vi "digital password.vi"() -> ()   [LabVIEW 2021]
panel:
  out "String":string
  out "String 3":string
  out "Password":string
  out "Slide":u8(slide) scale=0.0..100.0
  in  "Password":T1
  # "1"
  # "2"
  # "3"
  # "4"
  # "5"
  # "6"
  # "7"
  # "8"
  # "9"
  # "0"
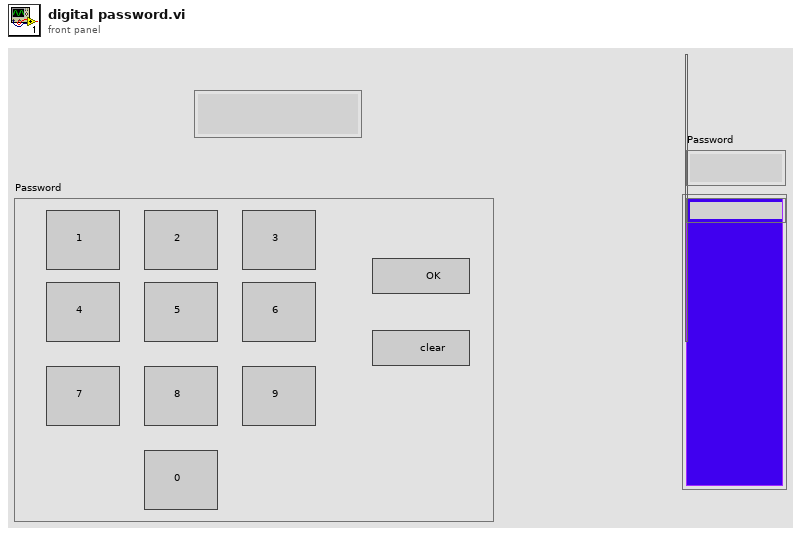
[diagram p1: front panel]
types:
  T1 = cluster{"Blank Button":bool, "Blank Button 2":bool, "Blank Button 3":bool, "Blank Button 4":bool, "Blank Button 5":bool, "Blank Button 6":bool, "Blank Button 7":bool, "Blank Button 8":bool, "Blank Button 9":bool, "Blank Button 10":bool, "OK Button":bool, "Refresh Button":bool}
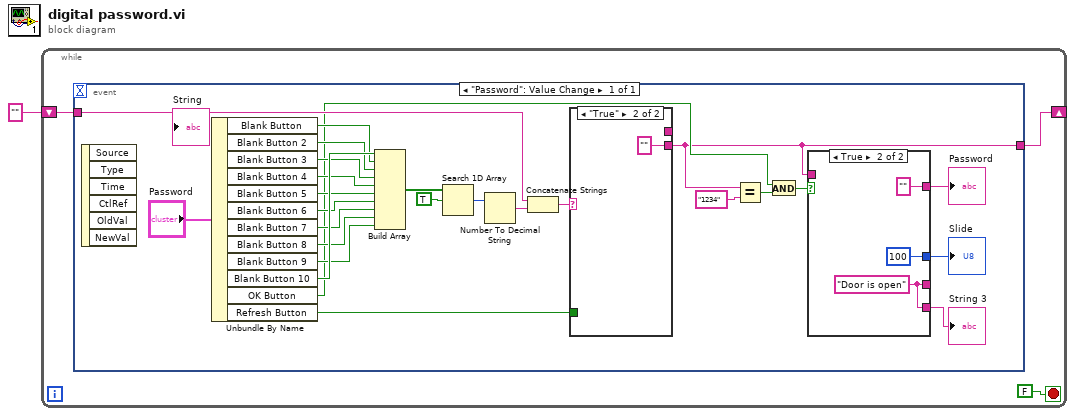
[diagram p0: block diagram]
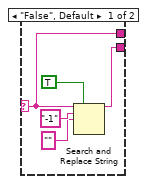
[diagram p2: hidden frame]
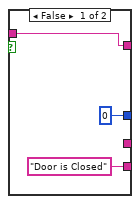
[diagram p3: hidden frame]
diagram:
  n1 = while {
    shift-right: [w3] -> _
    shift-left: "" -> [w2]
    stop <- FALSE stop-if-true
    n2 = event shown="[0] \"Password\": Value Change" {
      selector: _ -> [_]
      dyn-events: _ -> [_]
      timeout: _ -> [_]
      tunnel: [w5] -> w3
      tunnel: w2 -> [w15]
      event "Password": Value Change {
        n3 = event-data() -> ()  [unwired: 1 in, 6 out]
        n4 = Unbundle By Name("Password") -> ("Blank Button"=w28:bool, "Blank Button 2"=w27:bool, "Blank Button 3"=w26:bool, "Blank Button 4"=w25:bool, "Blank Button 5"=w24:bool, "Blank Button 6"=w23:bool, "Blank Button 7"=w22:bool, "Blank Button 8"=w21:bool, "Blank Button 9"=w20:bool, "Blank Button 10"=w29:bool, "OK Button"=w11:bool, "Refresh Button"=w7:bool)
        n5 = Build Array(w29, w28, w27, w26, w25, w24, w23, w22, w21, w20) -> (w18:bool[])
        n6 = Search 1D Array(1D array=w18, element=TRUE) -> (index of element=w19:i32)  [unwired: 1 in]
        n7 = Number To Decimal String(number=w19) -> (decimal integer string=w16:string)  [unwired: 1 in]
        n8 = Concatenate Strings(w15, w16) -> (w8:string)
        n9 = case shown="\"True\"" w8 {
          selector: w8 -> [w31 _]
          tunnel: [w31 _] -> _
          tunnel: [w32 "" ("result string")] -> w5
          tunnel: w7 -> [_ _]
          frame "False", Default {
            n10 = Search and Replace String(replace all?=TRUE ("replace all? (F)"), input string=w31, search string="-1", replace string="" ("replace string (\"\")")) -> (result string=w32:string)  [unwired: 4 in, 3 out]
          }
          frame "True" {
          }
        }
        n11 = Equal?(x=w5, y="1234") -> (x = y?=w10:bool)
        n12 = And(x=w11, y=w10) -> (x .and. y?=w9:bool)
        n13 = case shown="True" w9 {
          tunnel: [u8 0 ("Slide") u8 100 ("Slide")] -> w13
          tunnel: [_ w41] -> _
          tunnel: ["Door is Closed" ("String 3") w41] -> w12
          tunnel: w5 -> [w37 _]
          tunnel: [w37 "" ("Password")] -> w6
          frame False {
          }
          frame True {
            w41 = "Door is open" ("String 3")
          }
        }
        "Password" <- w6
        "Slide" <- w13
        "String 3" <- w12
      }
    }
  }
